vi "Dataset Transaction Id 2 Label.vi"(10 "Dataset Trans Id":T1) -> (2 "Label":string)   [LabVIEW 2009]
uses:
  Dataset Transaction Id.ctl
  Dataset Source.ctl
  Dataset Type.ctl
  Apps/Yes No Button.ctl
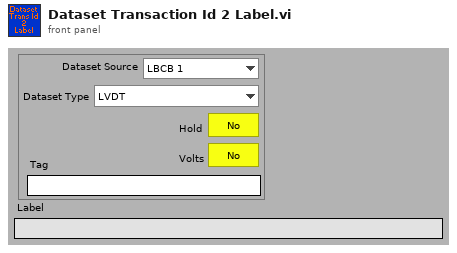
[diagram p1: front panel]
types:
  T1 = typedef "Dataset Transaction Id.ctl" = cluster{"Dataset Source":T2, "Dataset Type":T3, "Hold":T4, "Volts":T4, "Tag":string}
  T2 = typedef "Dataset Source.ctl" = enum16{"LBCB 1", "LBCB 2", "Combined", "External Sensors"}
  T3 = typedef "Dataset Type.ctl" = enum16{"LVDT", "Load Cell", "Actuator Command", "Servo Error", "Displacement Command", "Displacement", "Force"}
  T4 = typedef "Yes No Button.ctl" = bool
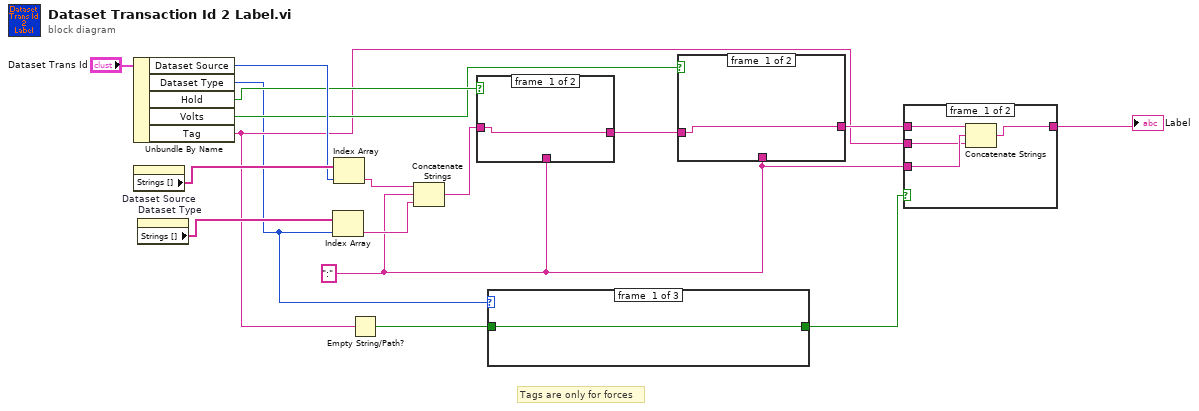
[diagram p0: block diagram]
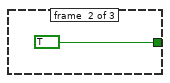
[diagram p2: hidden frame]
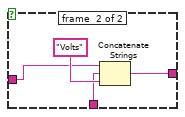
[diagram p5: hidden frame]
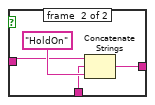
[diagram p6: hidden frame]
diagram:
  w5 = ":"
  # "Tags are only for forces"
  n1 = Unbundle By Name("Dataset Trans Id") -> ("Dataset Source"=w15:T2, "Dataset Type"=w3:T3, "Hold"=w11:T4, "Volts"=w10:T4, "Tag"=w4:string)
  n2 = property on="Dataset Source" class="Enum (strict)"() -> ("Strings []"=w16:string[])  [unwired: 2 in, 2 out]
  n3 = property on="Dataset Type" class="Enum (strict)"() -> ("Strings []"=w14:string[])  [unwired: 2 in, 2 out]
  n4 = Index Array(array=w14, index=w3) -> (element=w12:string)
  n5 = Index Array(array=w16, index=w15) -> (element=w13:string)
  n6 = Empty String/Path?(string/path=w4) -> (empty?=w2:bool)
  n7 = Concatenate Strings(w13, w5, w12) -> (w9:string)
  n8 = case shown="True" w11 {
    tunnel: w9 -> [w18 w20]
    tunnel: w5 -> [_ w21]
    tunnel: [w18 w19] -> w8
    frame #0 {
    }
    frame #1 {
      n9 = Concatenate Strings(w20, w21, "HoldOn" ("string")) -> (w19:string)
    }
  }
  n10 = case shown="\"Actuator Command\", Default" w3 {
    tunnel: w2 -> [w23 _ w25]
    tunnel: [w23 TRUE w25] -> w1
    frame #0 {
    }
    frame #1 {
    }
    frame #2 {
    }
  }
  n11 = case shown="True" w10 {
    tunnel: w8 -> [w26 w29]
    tunnel: w5 -> [_ w28]
    tunnel: [w26 w27] -> w7
    frame #0 {
    }
    frame #1 {
      n12 = Concatenate Strings(w29, w28, "Volts" ("string")) -> (w27:string)
    }
  }
  n13 = case shown="True" w1 {
    tunnel: w7 -> [w34 w35]
    tunnel: [w33 w35] -> w6
    tunnel: w5 -> [w32 _]
    tunnel: w4 -> [w31 _]
    frame #0 {
      n14 = Concatenate Strings(w34, w32, w31) -> (w33:string)
    }
    frame #1 {
    }
  }
  "Label" <- w6
